vi "Reset Meter Properties.vi"(8 "error in (no error)":errorcluster, 11 "VISA resource name":refnum<visa-resource-name>) -> (0 "error out":errorcluster, 3 "VISA resource name out":refnum<visa-resource-name>)   [LabVIEW 2015, in "Fluke 289.lvlib"]
doc: "Resets meter properties to their factory default state."
uses:
  <instrlib>/Fluke 289/Fluke 289.lvlib
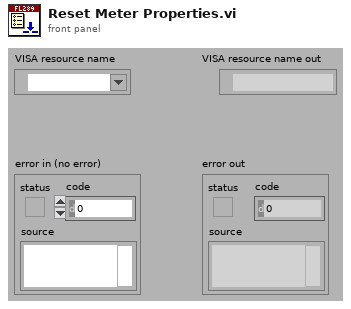
[diagram p1: front panel]
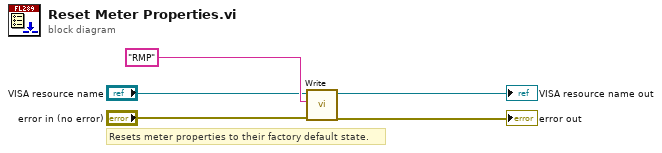
[diagram p0: block diagram]
diagram:
  # "Resets meter properties to their factory default state."
  n1 = call <instrlib>:"Write.vi"("error in (no error)"="error in (no error)", "Write Buffer"="RMP", "VISA resource name"="VISA resource name") -> ("error out"=→"error out":errorcluster, "VISA resource name out"=→"VISA resource name out":refnum<visa-resource-name>)  [unwired: 7 in]
